vi "Get SMO Port.vi"(8 "error in (no error)":errorcluster, 11 "Inst.MagnetoInstrument in":refnum<class "Inst.Magneto.lvclass">) -> (0 "error out":errorcluster, 2 "Port":u16, 3 "Inst.MagnetoInstrument out":refnum<class "Inst.Magneto.lvclass">)   [LabVIEW 2019, in "Inst.Magneto.lvclass"]
uses:
  Inst.Magneto.lvclass
  <userlib>/Levylab/Instrument Framework/Instrument Types/VSource/Instrument.VSource.lvclass
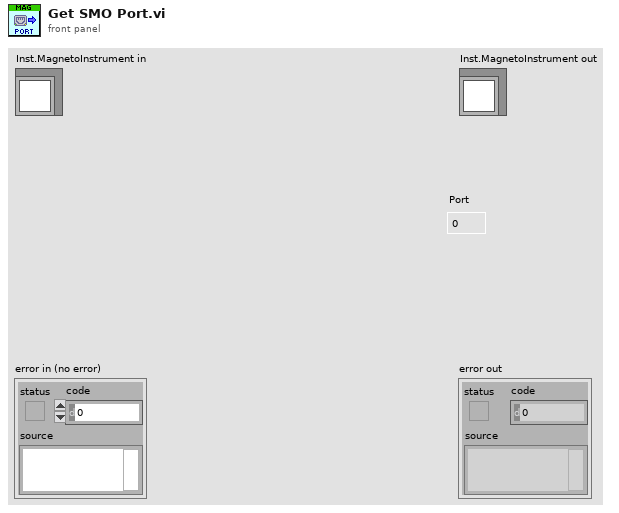
[diagram p1: front panel]
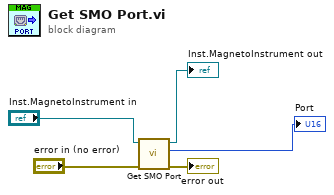
[diagram p0: block diagram]
diagram:
  n1 = call-parent "Get SMO Port.vi"("error in (no error)"="error in (no error)", "Instrument in"="Inst.MagnetoInstrument in") -> ("error out"=→"error out":errorcluster, "Port"=→"Port":u16, "Instrument out"=→"Inst.MagnetoInstrument out":refnum<class "Inst.Magneto.lvclass">)  [unwired: 7 in]
